vi "Write_Protection_Global.vi"() -> ()   [LabVIEW 2016, in "CS++Actor.lvlib" / "CS++Actor.lvclass"]
uses:
  CS++Actor.lvclass
panel:
  in  "WriteProtectedMessages":string[](array[string])
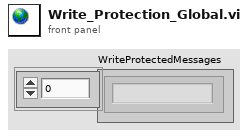
[diagram p1: front panel]
diagram:
